vi "Get Audio In (SubVI).vi"(8 "error in (no error)":errorcluster, 11 "Refnum in":T1) -> (0 "error out":errorcluster, 1 "Right Audio In":i16[](array[numeric]), 2 "Left Audio In":i16[](array[numeric]), 3 "Refnum out":T1)   [LabVIEW 2014]
uses:
  Controls/FPGA Reference.ctl
  Controls/sample block size.vi
  <vilib>/Utility/error.llb/Error Cluster From Error Code.vi
  <vilib>/rvi/errors/niLvFpgaAdjustHostInterfaceError.vi
  <vilib>/rvi/interface/nirviMethod/nirviMethod.xnode
  <vilib>/FPGAPlugInAG/Dynamic/niLvFpga_ReadFifo_Dynamic.vi
  <vilib>/rvi/errors/niLvFpgaMergeErrorWithErrorCode.vi
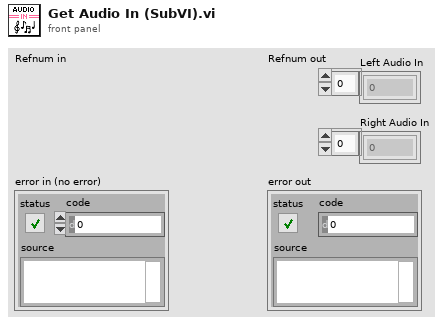
[diagram p1: front panel]
types:
  T1 = typedef "FPGA Reference.ctl" = refnum<k20>
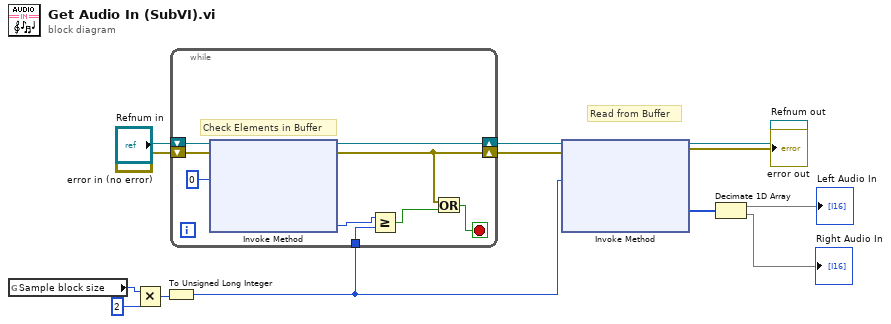
[diagram p0: block diagram]
diagram:
  # "Read from Buffer"
  n1 = global read "sample block size.vi" "Sample block size"() -> (w4:i32)
  n2 = Multiply(x=w4, y=2) -> (x*y=w2:i32)
  n3 = To Unsigned Long Integer(number=w2) -> (unsigned 32bit integer=w1:u32)
  n4 = while {
    shift-right: [w22] -> w11
    shift-left: "Refnum in" -> [w20]
    shift-right: [w17] -> w8
    shift-left: "error in (no error)" -> [w19]
    tunnel: w1 -> [w14]
    stop <- w15 stop-if-true
    # "Check Elements in Buffer"
    n5 = xnode "Invoke Method"("FPGA VI Reference In"=w20, "error in"=w19, "Number of Elements"=u32 0) -> ("FPGA VI Reference Out"=w22:T1, "error out"=w17:errorcluster, "Elements Remaining"=w18:u32)  [unwired: 1 in, 1 out]
    n6 = Greater Or Equal?(x=w18, y=w14) -> (x >= y?=w16:bool)
    n7 = Or(x=w17, y=w16) -> (x .or. y?=w15:bool)
  }
  n8 = xnode "Invoke Method"("FPGA VI Reference In"=w11, "error in"=w8, "Number of Elements"=w1) -> ("FPGA VI Reference Out"=→"Refnum out":T1, "error out"=→"error out":errorcluster, "Data"=w7:i16[])  [unwired: 1 in, 1 out]
  n9 = Decimate 1D Array(w7) -> (→"Left Audio In":i16[], →"Right Audio In":i16[])
